vi "Draw.vi"(0 "picture in":picture, 5 "Display State":T1, 11 "error in (no error)":errorcluster) -> (4 "picture out":picture)   [LabVIEW 2015, in "FSM Editor.xctl"]
uses:
  FSM Editor.xctl
  State.vi
  Classes/FSM.Port/FSM.Port.lvclass
  <vilib>/Utility/miscctls.llb/LVPoint32TypeDef.ctl
  Drag Mode.ctl
  Events.ctl
  NodeAdded.ctl
  NodeSelected.ctl
  EdgeEventData.ctl
  Classes/FSM.Port/FSM.Port.lvclass/FSM.Port.ctl
  Classes/FSM.Port/Read Location.vi
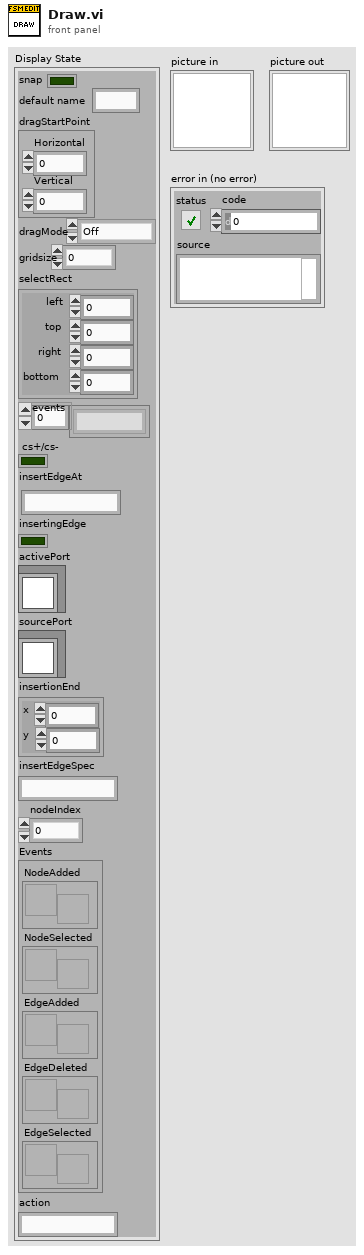
[diagram p1: front panel]
types:
  T1 = typedef "FSM Editor.xctl/State.vi" = cluster{"snap":bool, "default name":string, "dragStartPoint":T2, "dragMode":T3, "gridsize":dbl, "selectRect":cluster{"left":i16, "top":i16, "right":i16, "bottom":i16}, "events":string[], "cs+/cs-":bool, "insertEdgeAt":string, "insertingEdge":bool, "activePort":refnum<class "FSM.Port.lvclass">, "sourcePort":refnum<class "FSM.Port.lvclass">, "insertionEnd":cluster{"x":i16, "y":i16}, "insertEdgeSpec":string, "nodeIndex":i32, "Events":T4, "action":string}
  T2 = typedef "LVPoint32TypeDef.ctl" = cluster{"Horizontal":i32, "Vertical":i32}
  T3 = typedef "Drag Mode.ctl" = enum16{"Off", "NodePending", "Nodes", "Pan", "Select", "EdgeInsertion", "EdgePoint", "EdgeLabel"}
  T4 = typedef "FSM Editor.xctl/Events.ctl" = cluster{"NodeAdded":refnum<user-event>, "NodeSelected":refnum<user-event>, "EdgeAdded":refnum<user-event>, "EdgeDeleted":refnum<user-event>, "EdgeSelected":refnum<user-event>}
  T5 = cluster{"left":i16, "top":i16, "right":i16, "bottom":i16}
  T6 = cluster{"Width":i16, "Style":enum32{"Solid", "Dash", "Dot", "DashDot", "DashDotDot"}}
  T7 = cluster{"Width":u16, "Style":enum32{"Solid", "Dash", "Dot", "DashDot", "DashDotDot"}}
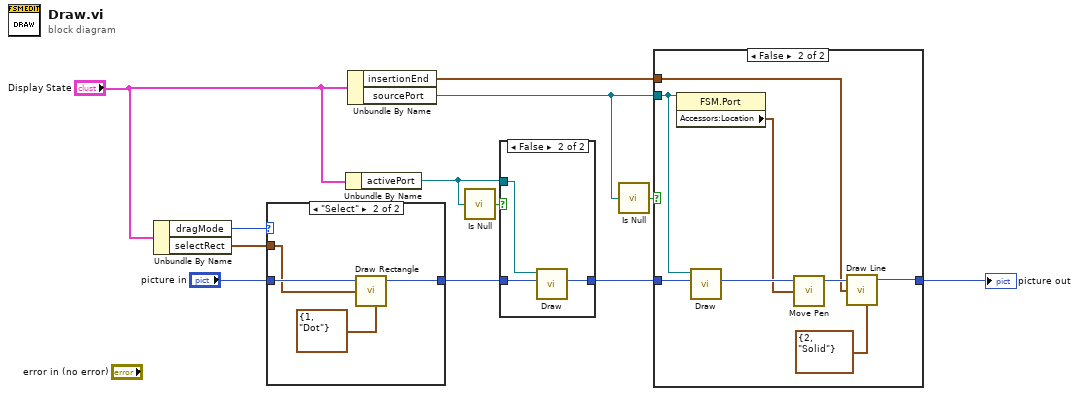
[diagram p0: block diagram]
diagram:
  n1 = Unbundle By Name("Display State") -> ("dragMode"=w12:T3, "selectRect"=w11:T5)
  n2 = case shown="\"Select\"" w12 {
    tunnel: w11 -> [_ w16]
    tunnel: "picture in" -> [w13 w17]
    tunnel: [w13 w14] -> w9
    frame "Off", Default {
    }
    frame "Select" {
      n3 = call <vilib>:"Draw Rectangle.vi"("picture"=w17, "rect"=w16, "pen"=T6 {"Width"=1, "Style"=enum."Dot"}) -> ("new picture"=w14:picture)  [unwired: 6 in]
    }
  }
  n4 = Unbundle By Name("Display State") -> ("activePort"=w8:refnum<class "FSM.Port.lvclass">)
  n5 = Unbundle By Name("Display State") -> ("insertionEnd"=w2:cluster{"x":i16, "y":i16}, "sourcePort"=w4:refnum<class "FSM.Port.lvclass">)
  n6 = call "Is Null.vi"("Port"=w8) -> ("null"=w7:bool)
  n7 = case shown="False" w7 {
    tunnel: w9 -> [w18 w21]
    tunnel: [w18 w20] -> w6
    tunnel: w8 -> [_ w19]
    frame True {
    }
    frame False {
      n8 = call "Draw.vi"("picture in"=w21, "Port in"=w19) -> ("picture out"=w20:picture)  [unwired: 7 in, 2 out]
    }
  }
  n9 = call "Is Null.vi"("Port"=w4) -> ("null"=w3:bool)
  n10 = case shown="False" w3 {
    tunnel: w6 -> [w22 w30]
    tunnel: [w22 w26] -> w1
    tunnel: w4 -> [_ w24]
    tunnel: w2 -> [_ w27]
    frame True {
    }
    frame False {
      n11 = property class="FSM.Port"(reference=w24) -> ("Accessors:Location"=w23:cluster{"x":i16, "y":i16})  [unwired: 1 in, 2 out]
      n12 = call "Draw.vi"("picture in"=w30, "Port in"=w24) -> ("picture out"=w29:picture)  [unwired: 7 in, 2 out]
      n13 = call <vilib>:"Move Pen.vi"("new position"=w23, "picture"=w29) -> ("new picture"=w28:picture)  [unwired: 3 in]
      n14 = call <vilib>:"Draw Line.vi"("picture"=w28, "end point"=w27, "pen"=T7 {"Width"=2, "Style"=enum."Solid"}) -> ("new picture"=w26:picture)  [unwired: 6 in]
    }
  }
  "picture out" <- w1
